vi "adjust_histogram_cursor.vi"(8 "error in (no error)":errorcluster, 10 "lock to bin edges":bool, 11 "histogram":refnum<vi>) -> (0 "error out":errorcluster, 3 "histogram out":refnum<vi>)   [LabVIEW 2019, in "graph_utilities.lvclass"]
uses:
  graph_utilities.lvclass
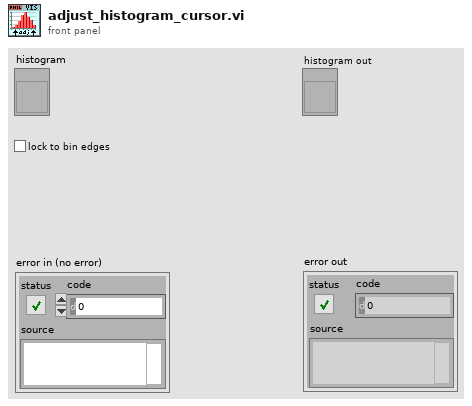
[diagram p1: front panel]
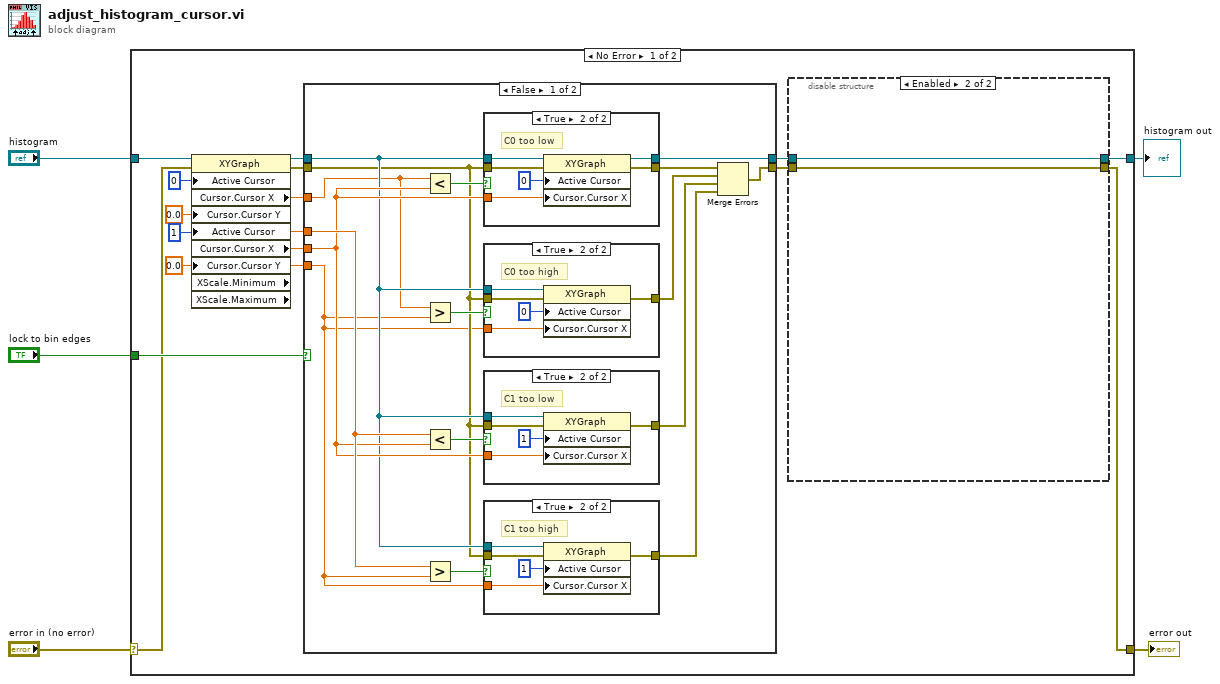
[diagram p0: block diagram]
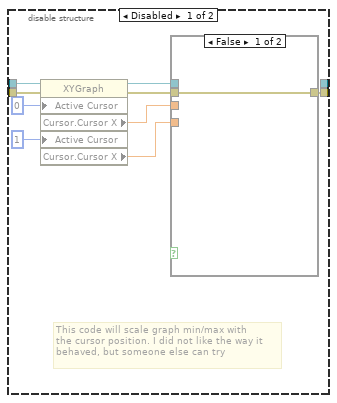
[diagram p2: hidden frame]
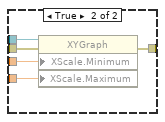
[diagram p3: hidden frame]
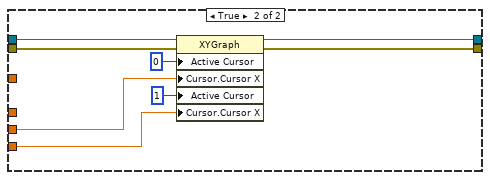
[diagram p8: hidden frame]
diagram:
  n1 = case shown="No Error" "error in (no error)" {
    selector: "error in (no error)" -> [w12 w91]
    tunnel: "lock to bin edges" -> [w16 _]
    tunnel: "histogram" -> [w15 w90]
    tunnel: [w9 w91] -> w3
    tunnel: [w6 w90] -> w1
    frame No Error {
      n2 = property on="Property Node" class="XYGraph"(reference=w15, error in=w12, "Active Cursor"=0, "Cursor.Cursor Y"=0.0 ("Cursor.Cursor Position:Cursor Y"), "Active Cursor"=1, "Cursor.Cursor Y"=0.0 ("Cursor.Cursor Position:Cursor Y")) -> (reference out=w14:refnum<vi>, error out=w13:errorcluster, "Cursor.Cursor X"=w20:dbl, "Cursor.Cursor X"=w19:dbl, "XScale.Minimum"=w18:dbl, "XScale.Maximum"=w17:dbl)
      n3 = case shown="False" w16 {
        tunnel: w20 -> [w42 _]
        tunnel: w19 -> [w51 _]
        tunnel: w18 -> [w50 w89]
        tunnel: w17 -> [w43 w87]
        tunnel: w14 -> [w49 w88]
        tunnel: w13 -> [w48 w86]
        tunnel: [w40 w85] -> w10
        tunnel: [w41 w82] -> w11
        frame False {
          n4 = Less?(x=w42, y=w50) -> (x < y?=w55:bool)
          n5 = Greater?(x=w42, y=w43) -> (0:w54:bool)
          n6 = Less?(x=w51, y=w50) -> (x < y?=w53:bool)
          n7 = Greater?(x=w51, y=w43) -> (0:w52:bool)
          n8 = case shown="True" w55 {
            tunnel: w49 -> [w74 w80]
            tunnel: w50 -> [_ w79]
            tunnel: w48 -> [w75 w78]
            tunnel: [w75 w77] -> w47
            tunnel: [w74 w76] -> w41
            frame False {
            }
            frame True {
              # "C0 too low"
              n9 = property on="Property Node" class="XYGraph"(reference=w80, error in=w78, "Active Cursor"=0, "Cursor.Cursor X"=w79) -> (reference out=w76:refnum<vi>, error out=w77:errorcluster)
            }
          }
          n10 = case shown="True" w54 {
            tunnel: w49 -> [_ w72]
            tunnel: w43 -> [_ w71]
            tunnel: w48 -> [w68 w70]
            tunnel: [w68 w69] -> w46
            frame False {
            }
            frame True {
              # "C0 too high"
              n11 = property on="Property Node" class="XYGraph"(reference=w72, error in=w70, "Active Cursor"=0, "Cursor.Cursor X"=w71) -> (error out=w69:errorcluster)  [unwired: 1 out]
            }
          }
          n12 = case shown="True" w53 {
            tunnel: w49 -> [_ w66]
            tunnel: w50 -> [_ w65]
            tunnel: w48 -> [w62 w64]
            tunnel: [w62 w63] -> w45
            frame False {
            }
            frame True {
              # "C1 too low"
              n13 = property on="Property Node" class="XYGraph"(reference=w66, error in=w64, "Active Cursor"=1, "Cursor.Cursor X"=w65) -> (error out=w63:errorcluster)  [unwired: 1 out]
            }
          }
          n14 = case shown="True" w52 {
            tunnel: w49 -> [_ w60]
            tunnel: w43 -> [_ w59]
            tunnel: w48 -> [w56 w58]
            tunnel: [w56 w57] -> w44
            frame False {
            }
            frame True {
              # "C1 too high"
              n15 = property on="Property Node" class="XYGraph"(reference=w60, error in=w58, "Active Cursor"=1, "Cursor.Cursor X"=w59) -> (error out=w57:errorcluster)  [unwired: 1 out]
            }
          }
          n16 = Merge Errors(w47, w46, w45, w44) -> (w40:errorcluster)
        }
        frame True {
          n17 = property on="Property Node" class="XYGraph"(reference=w88, error in=w86, "Active Cursor"=0, "Cursor.Cursor X"=w89, "Active Cursor"=1, "Cursor.Cursor X"=w87) -> (reference out=w82:refnum<vi>, error out=w85:errorcluster)
        }
      }
      n18 = disable-structure shown="Enabled" {
        disable-tunnel: w11 -> [w29 w38]
        disable-tunnel: w10 -> [w28 w39]
        disable-tunnel: [w23 w39] -> w9
        disable-tunnel: [_ w38] -> w6
        frame Disabled {
          # "This code will scale graph min/max with\nthe cursor position. I did not like the way it\nbehaved, but someone else can try"
          n19 = property on="Property Node" class="XYGraph"(reference=w29, error in=w28, "Active Cursor"=0, "Active Cursor"=1) -> (reference out=w27:refnum<vi>, error out=w26:errorcluster, "Cursor.Cursor X"=w25:dbl, "Cursor.Cursor X"=w24:dbl)
          n20 = case shown="False" {
            selector: _ -> [_ _]
            tunnel: w27 -> [_ w37]
            tunnel: w26 -> [w32 w36]
            tunnel: [w32 w35] -> w23
            tunnel: w25 -> [_ w34]
            tunnel: w24 -> [_ w33]
            frame False {
            }
            frame True {
              n21 = property on="Property Node" class="XYGraph"(reference=w37, error in=w36, "XScale.Minimum"=w34, "XScale.Maximum"=w33) -> (error out=w35:errorcluster)  [unwired: 1 out]
            }
          }
        }
        frame Enabled {
        }
      }
    }
    frame Error {
    }
  }
  "error out" <- w3
  "histogram out" <- w1
